vi "S7-TCP_Demo.vi"() -> ()   [LabVIEW 2018]
uses:
  S7-TCP/Controls/WriteDataType.ctl
  S7-TCP/S7-TCP.lvclass
  S7-TCP/Controls/RegisterType.ctl
panel:
  out "WriteData Valid":bool
  in  "WriteData":sgl[](array[numeric])
  in  "WriteAddress":sgl format="%#.1g"
  in  "DataType":T1
  in  "WriteDB Block":u16=600
  out "ReadDataValid":bool
  out "ReadData":u8[](array[numeric])
  in  "ReadDB Block":u16=600
  in  "ReadLength":u16=1
  in  "ReadStartAddress":u32
  in  "Write":bool
  in  "read":bool
  in  "PLC":u8(ring) items=["S7-1200.200SMART"=0, "S7-300"=2, "S7-400"=3]
  in  "IP Address":string="192.168.6.10"
  out "time":u32
  in  "停止":bool
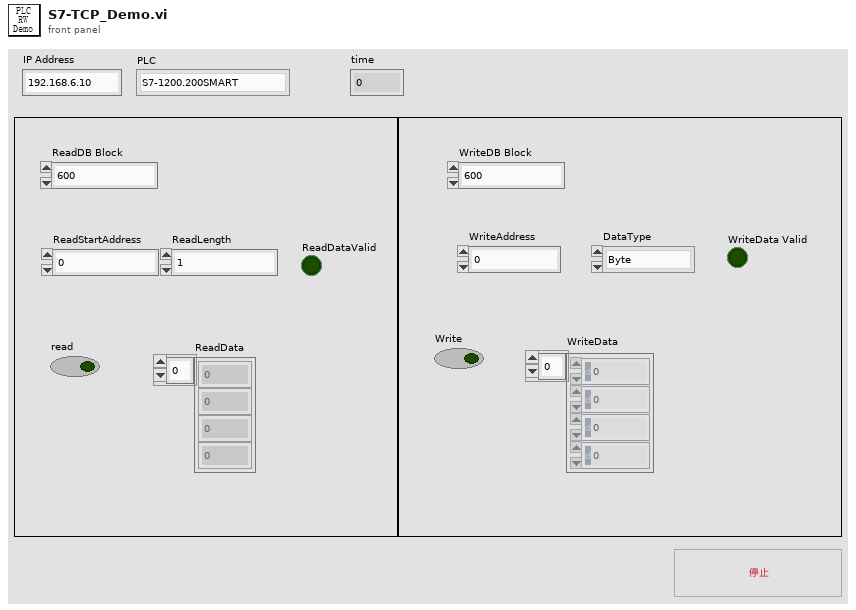
[diagram p1: front panel]
types:
  T1 = typedef "S7-TCP.lvclass/WriteDataType.ctl" = enum16{"Byte", "Word", "Dword", "Real", "Bit"}
  T2 = typedef "S7-TCP.lvclass/RegisterType.ctl" = u8
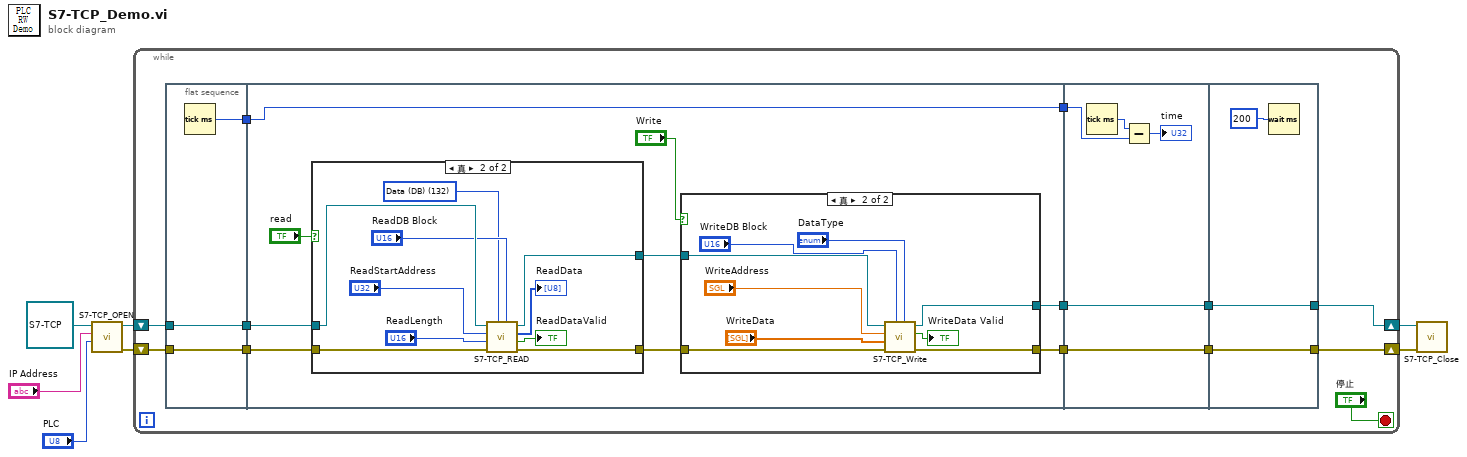
[diagram p0: block diagram]
diagram:
  n1 = call "S7-TCP_OPEN.vi"("PLC"="PLC", "IP Address"="IP Address", "S7-TCP 输入"=refnum<class "S7-TCP.lvclass"> refnum) -> ("error out"=w4:errorcluster, "S7-TCP 输出"=w3:refnum<class "S7-TCP.lvclass">)  [unwired: 6 in, 1 out]
  n2 = while {
    shift-right: [w14] -> w2
    shift-left: w4 -> [w15]
    shift-right: [w11] -> w1
    shift-left: w3 -> [w17]
    stop <- "停止" stop-if-true
    n3 = flat-sequence {
      tunnel: [w23] -> w20
      tunnel: [w22] -> w18
      tunnel: w17 -> [w22]
      tunnel: [w21] -> w16
      tunnel: w15 -> [w21]
      tunnel: w20 -> [w32]
      tunnel: [w32] -> w19
      tunnel: w18 -> [w31]
      tunnel: w16 -> [w28]
      tunnel: [w25] -> w12
      tunnel: [w24] -> w9
      tunnel: w19 -> [w59]
      tunnel: [w57] -> w13
      tunnel: w12 -> [w57]
      tunnel: [w56] -> w10
      tunnel: w9 -> [w56]
      tunnel: [w62] -> w14
      tunnel: w13 -> [w62]
      tunnel: [w61] -> w11
      tunnel: w10 -> [w61]
      frame #0 {
        n4 = Tick Count (ms)() -> (millisecond timer value=w23:u32)
      }
      frame #1 {
        n5 = case shown="真" "read" {
          tunnel: w31 -> [w45 w55]
          tunnel: [w45 w54] -> w29
          tunnel: w28 -> [w44 w53]
          tunnel: [w44 w52] -> w26
          frame False {
          }
          frame True {
            w46 = T2 132 items=["I/O (P)"=128, "Input (I)"=129, "Output (Q)"=130, "Bit Memory (M)"=131, "Data (DB)"=132, "Instance Data (DI)"=133, "Local Data (L)"=134, "Predecessor Local Data (VL)"=135] ("RegisterType")
            n6 = call "S7-TCP_READ.vi"("DB Block"="ReadDB Block", "RegisterType"=w46, "error in (no error)"=w53, "Length"="ReadLength", "StartAddress"="ReadStartAddress", "S7-TCP 输入"=w55) -> ("error out"=w52:errorcluster, "DataValid"=→"ReadDataValid":bool, "ReadData"=→"ReadData":u8[], "S7-TCP 输出"=w54:refnum<class "S7-TCP.lvclass">)  [unwired: 2 in]
          }
        }
        n7 = case shown="真" "Write" {
          tunnel: w29 -> [w34 w40]
          tunnel: w26 -> [w33 w43]
          tunnel: [w33 w42] -> w25
          tunnel: [w34 w41] -> w24
          frame False {
          }
          frame True {
            n8 = call "S7-TCP_Write.vi"("DataType"="DataType", "DB #"="WriteDB Block", "error in (no error)"=w43, "WriteData"="WriteData", "WriteAddress"="WriteAddress", "S7-TCP 输入"=w40) -> ("error out"=w42:errorcluster, "Data Valid"=→"WriteData Valid":bool, "S7-TCP 输出"=w41:refnum<class "S7-TCP.lvclass">)  [unwired: 3 in]
          }
        }
      }
      frame #2 {
        n9 = Tick Count (ms)() -> (millisecond timer value=w60:u32)
        n10 = Subtract(x=w60, y=w59) -> (x-y=→"time":u32)
      }
      frame #3 {
        n11 = Wait (ms)(milliseconds to wait=u32 200 ("等待时间（毫秒）")) -> ()  [unwired: 1 out]
      }
    }
  }
  n12 = call "S7-TCP_Close.vi"("error in (no error)"=w2, "S7-TCP 输入"=w1) -> ()  [unwired: 9 in, 1 out]
